vi "GB_DCIR.vi"(8 "errin":errorcluster, 10 "SN":string, 11 "L2T 2":T1 caption="Limites de test pris en compte") -> (0 "errout":errorcluster)   [LabVIEW 2020]
uses:
  Ctrl/L2T.ctl
  1d7331e3-373a-49af-a43b-51add20e1a94.vi
  VarGLO/Global PEAK.vi
  02 SLIM ZEN WS 500/SubVi/VG_progressBar.vi
  <instrlib>/IT6000C/IT6000C.lvlib
panel:
  out "PLC requet":string
  out "RDCIR":dbl
  # "Pre DCIR_____________________________________"
  # "intra DCIR_____________________________________"
  # "Post DCIR_____________________________________"
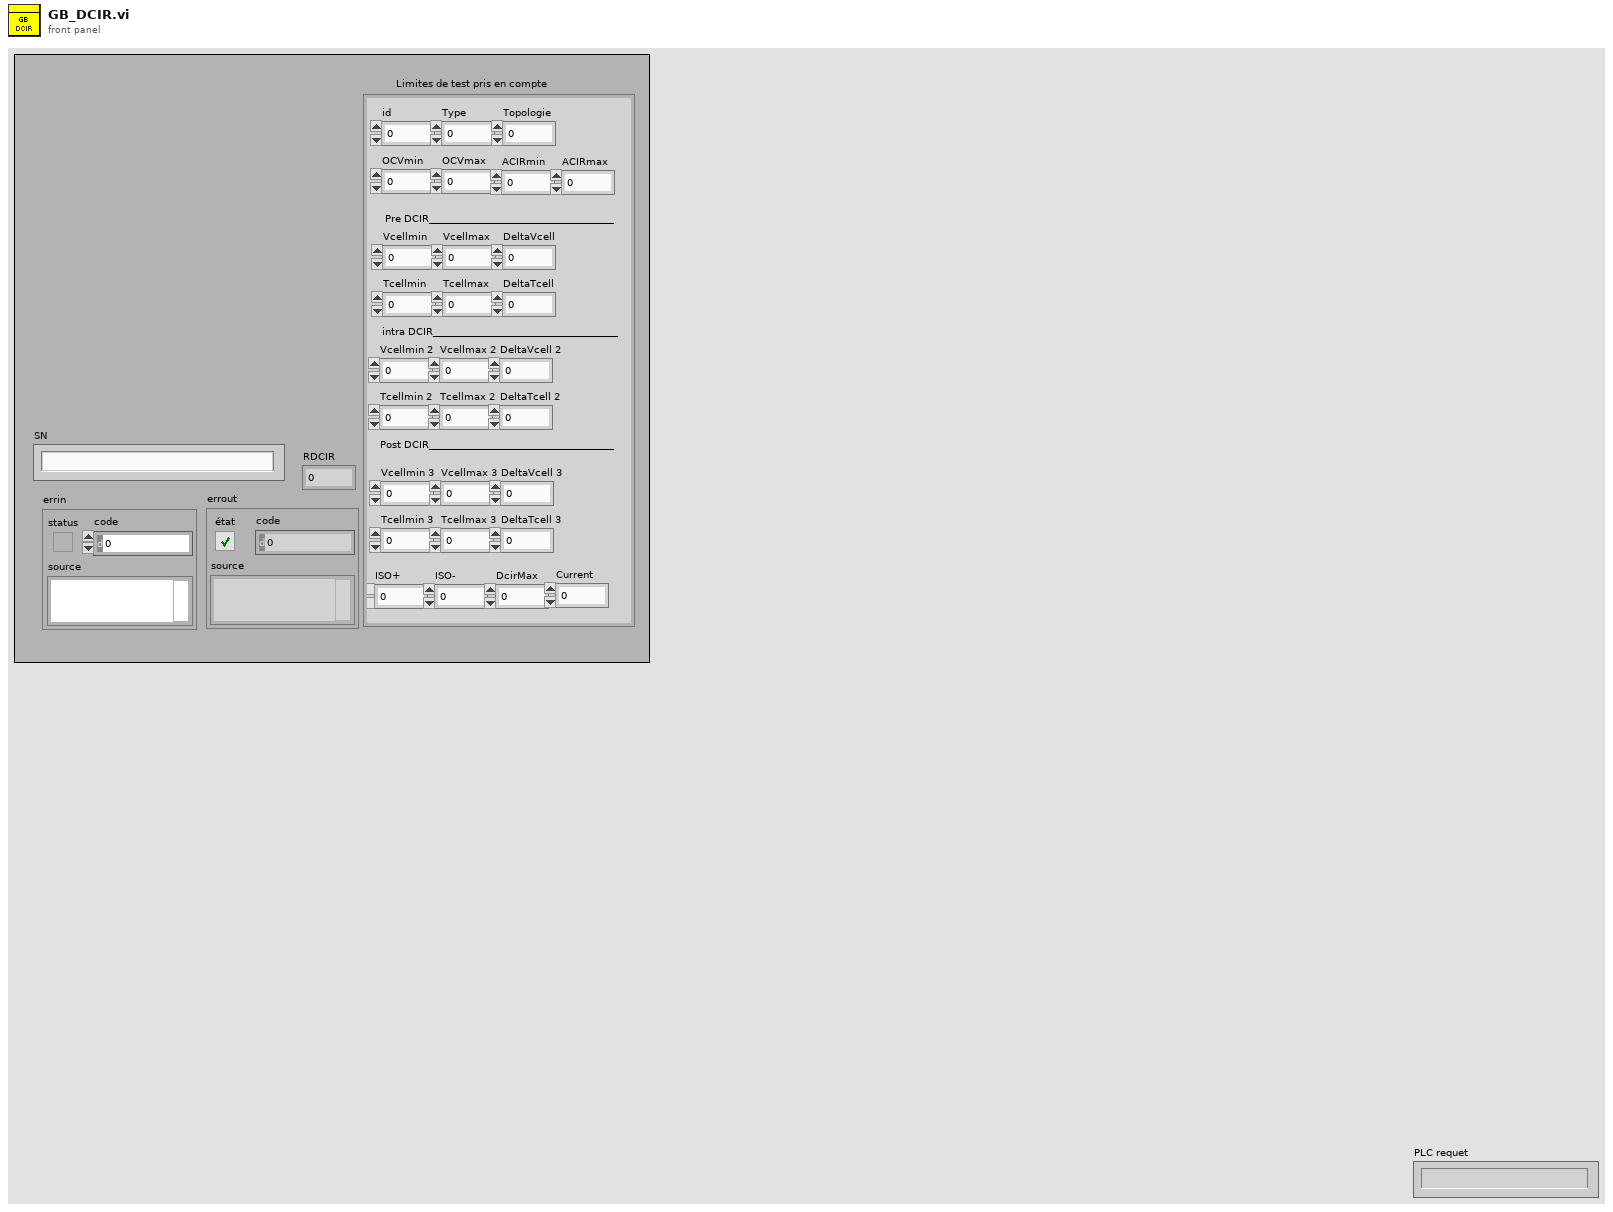
[diagram p1: front panel]
types:
  T1 = typedef "L2T.ctl" = cluster{"id":dbl, "Type":dbl, "OCVmin":dbl, "OCVmax":dbl, "ACIRmin":dbl, "ACIRmax":dbl, "Vcellmin":dbl, "Vcellmax":dbl, "DeltaVcell":dbl, "Tcellmin":dbl, "Tcellmax":dbl, "DeltaTcell":dbl, "ISO+":dbl, "ISO-":dbl, "DcirMax":dbl, "Current":dbl, "Topologie":dbl, "Vcellmin 2":dbl, "Vcellmax 2":dbl, "DeltaVcell 2":dbl, "Tcellmin 2":dbl, "Tcellmax 2":dbl, "DeltaTcell 2":dbl, "Vcellmin 3":dbl, "Vcellmax 3":dbl, "DeltaVcell 3":dbl, "Tcellmin 3":dbl, "Tcellmax 3":dbl, "DeltaTcell 3":dbl}
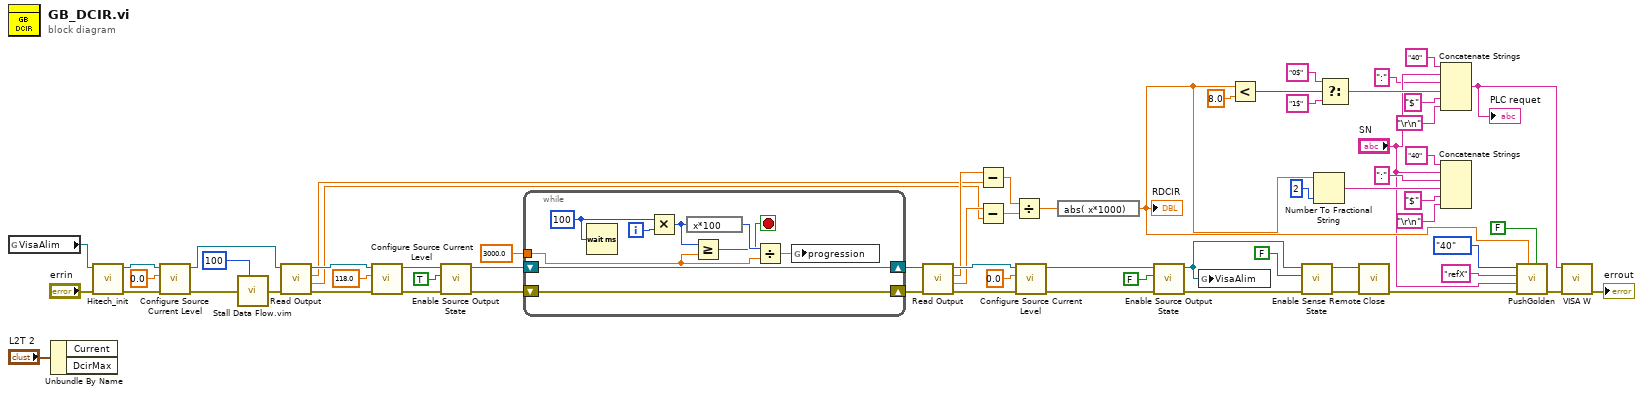
[diagram p0: block diagram]
diagram:
  n1 = global read "Global PEAK.vi" "VisaAlim"() -> (w32:refnum<visa-resource-name>)
  n2 = Unbundle By Name("L2T 2") -> ()  [unwired: 2 out]
  n3 = call "Hitech_init.vi"("errin"="errin", "VISA HITECH"=w32) -> ("error out"=w34:errorcluster, "VisaHitech"=w31:refnum<visa-resource-name>)  [unwired: 8 in]
  n4 = call <instrlib>:"Configure Source Current Level.vi"("error in (no error)"=w34, "Value(0)"=0.0, "VISA resource name"=w31) -> ("error out"=w37:errorcluster, "VISA resource name out"=w62:refnum<visa-resource-name>)  [unwired: 7 in]
  n5 = call "Stall Data Flow.vim"("value in"=w37, "milliseconds to wait"=u32 100) -> ("value out"=w36:errorcluster)  [unwired: 1 out]
  n6 = call <instrlib>:"Read Output.vi"("error in (no error)"=w36, "VISA resource name"=w62) -> ("error out"=w61:errorcluster, "Actual Current Level (A)"=w39:dbl, "Actual Voltage Level (V)"=w40:dbl, "VISA resource name out"=w60:refnum<visa-resource-name>)  [unwired: 6 in]
  n7 = call <instrlib>:"Configure Source Current Level.vi"("error in (no error)"=w61, "Value(0)"=118.0, "VISA resource name"=w60) -> ("error out"=w59:errorcluster, "VISA resource name out"=w58:refnum<visa-resource-name>)  [unwired: 7 in]
  n8 = call <instrlib>:"Enable Source Output State.vi"("error in (no error)"=w59, "Enable(True)"=TRUE, "VISA resource name"=w58) -> ("error out"=w54:errorcluster, "VISA resource name out"=w55:refnum<visa-resource-name>)  [unwired: 7 in]
  n9 = while {
    tunnel: sgl 3000.0 ("Ton") -> [w68]
    shift-right: [w66] -> w41
    shift-left: w55 -> [w66]
    shift-right: [w67] -> w42
    shift-left: w54 -> [w67]
    i -> [w72]
    stop <- w65 stop-if-true
    w71 = u32 100 ("attente (ms)")
    n10 = Wait (ms)(milliseconds to wait=w71) -> ()  [unwired: 1 out]
    n11 = Multiply(x=w71, y=w72) -> (x*y=w69:u32)
    n12 = expression code="x*100"(w69) -> (w70:u32)
    n13 = Greater Or Equal?(x=w69, y=w68) -> (x >= y?=w65:bool)
    n14 = Divide(x=w70, y=w68) -> (x/y=w64:sgl)
    n15 = global write "VG_progressBar.vi" "progression"(w64) -> ()
  }
  n16 = call <instrlib>:"Read Output.vi"("error in (no error)"=w42, "VISA resource name"=w41) -> ("error out"=w52:errorcluster, "Actual Current Level (A)"=w44:dbl, "Actual Voltage Level (V)"=w45:dbl, "VISA resource name out"=w51:refnum<visa-resource-name>)  [unwired: 6 in]
  n17 = Subtract(x=w45, y=w40) -> (x-y=w43:dbl)
  n18 = Subtract(x=w44, y=w39) -> (x-y=w47:dbl)
  n19 = Divide(x=w43, y=w47) -> (x/y=w46:dbl)
  n20 = call <instrlib>:"Configure Source Current Level.vi"("error in (no error)"=w52, "Value(0)"=0.0, "VISA resource name"=w51) -> ("error out"=w50:errorcluster, "VISA resource name out"=w49:refnum<visa-resource-name>)  [unwired: 7 in]
  n21 = expression code="abs( x*1000)"(w46) -> (w7:dbl)
  "RDCIR" <- w7
  n22 = call <instrlib>:"Enable Source Output State.vi"("error in (no error)"=w50, "Enable(True)"=FALSE, "VISA resource name"=w49) -> ("error out"=w16:errorcluster, "VISA resource name out"=w15:refnum<visa-resource-name>)  [unwired: 7 in]
  n23 = global write "Global PEAK.vi" "VisaAlim"(w15) -> ()
  n24 = Less?(x=w7, y=8.0) -> (x < y?=w5:bool)
  n25 = call <instrlib>:"Enable Sense Remote State.vi"("error in (no error)"=w16, "Enable(True)"=FALSE, "VISA resource name"=w15) -> ("error out"=w17:errorcluster, "VISA resource name out"=w14:refnum<visa-resource-name>)  [unwired: 7 in]
  n26 = Number To Fractional String(number=w7, precision (6)=i16 2) -> (F-format string=w25:string)  [unwired: 2 in]
  n27 = Select(t="0$" ("chaîne"), s=w5, f="1$" ("chaîne")) -> (s? t:f=w9:string)
  n28 = call <instrlib>:"Close.vi"("error in (no error)"=w17, "VISA resource name"=w14) -> ("error out"=w30:errorcluster)  [unwired: 9 in]
  n29 = Concatenate Strings("40" ("chaîne"), "SN", ":" ("string"), w9, "$" ("string"), "\r\n") -> (w1:string)
  "PLC requet" <- w1
  n30 = Concatenate Strings("40" ("chaîne"), "SN", ":" ("string"), w25, "$" ("string"), "\r\n") -> ()  [unwired: 1 out]
  n31 = call "PushGolden.vi"("isInt?"=FALSE, "Value"=w7, "errin"=w30, "SN"="SN", "refFile"="refX", "testnumber"=enum16{"50", "40", "30", "20", "11", "10", ""}."40") -> ("error out"=w21:errorcluster)  [unwired: 5 in]
  n32 = call "VISA W.vi"("errin"=w21, "Chaîne"=w1) -> ("errout"=→"errout":errorcluster)  [unwired: 9 in]
